vi "Convert-map-to-2D.vi"(8 "error in":errorcluster, 9 "Ycoords":sgl[](array[numeric]), 10 "Xcoords":sgl[](array[numeric]), 11 "Signal":dbl[](array[numeric])) -> (0 "error IO":errorcluster, 3 "2D map":dbl[][](array[numeric]))   [LabVIEW 2013, in "CameraVision.lvlib" / "CV-UI.lvclass"]
doc: "This function deletes the data from the various GUI graphs and displays. This avoids interference with data from a previous acquisition."
uses:
  CV-UI.lvclass
panel:
  out "Yscale":sgl
  out "Xscale":sgl
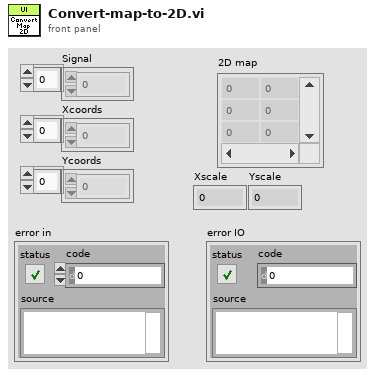
[diagram p1: front panel]
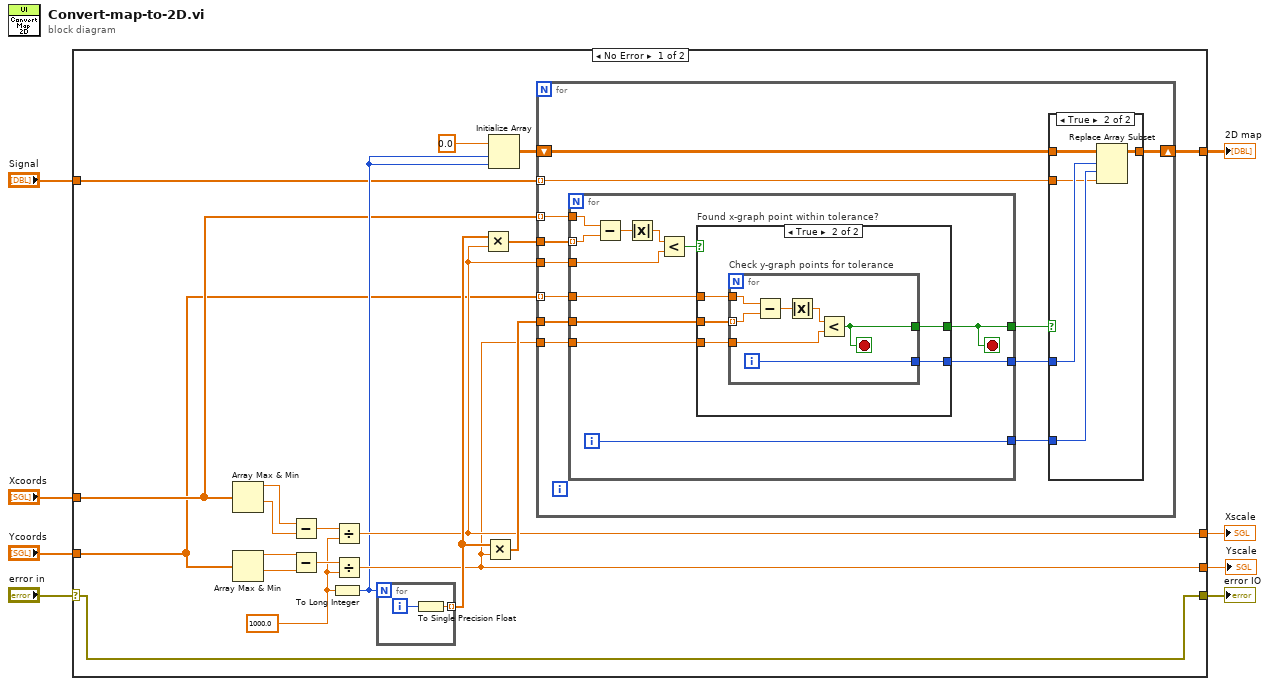
[diagram p0: block diagram]
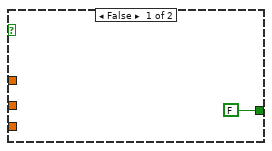
[diagram p3: hidden frame]
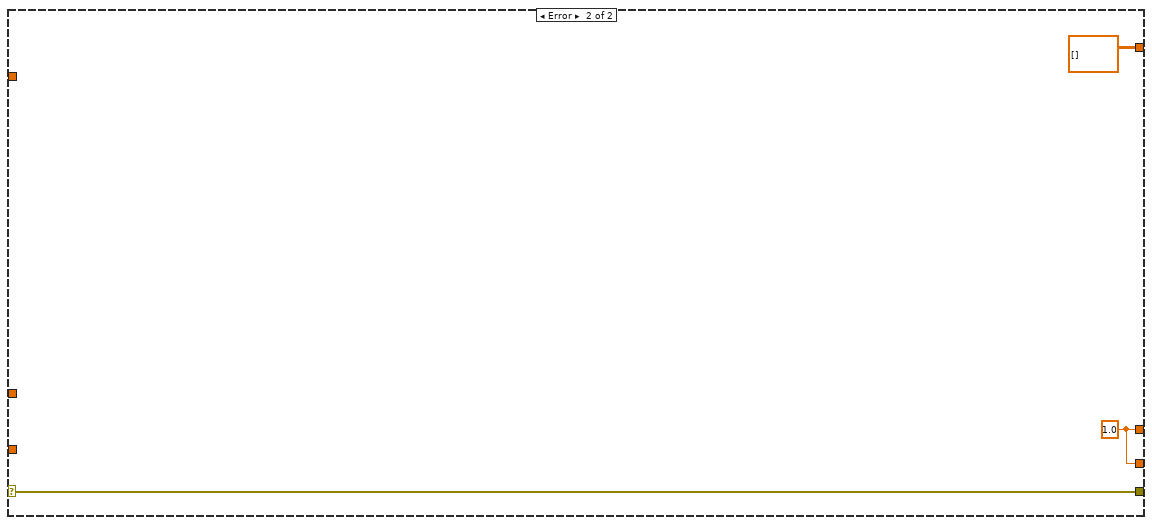
[diagram p4: hidden frame]
diagram:
  n1 = case shown="No Error" "error in" {
    selector: "error in" -> [w12 w76]
    tunnel: [w12 w76] -> w8
    tunnel: [w17 w75] -> w5
    tunnel: [w18 w75] -> w6
    tunnel: [w13 sgl[][] []] -> w4
    tunnel: "Xcoords" -> [w11 _]
    tunnel: "Ycoords" -> [w10 _]
    tunnel: "Signal" -> [w9 _]
    frame No Error {
      w22 = sgl 1000.0
      n2 = Array Max & Min(array=w11) -> (max value=w28:sgl, min value=w27:sgl)  [unwired: 2 out]
      n3 = Array Max & Min(array=w10) -> (max value=w24:sgl, min value=w23:sgl)  [unwired: 2 out]
      n4 = Subtract(x=w28, y=w27) -> (x-y=w25:sgl)
      n5 = Subtract(x=w24, y=w23) -> (x-y=w26:sgl)
      n6 = To Long Integer(number=w22) -> (32bit integer=w15:i32)
      n7 = Divide(x=w25, y=w22) -> (x/y=w18:sgl)
      n8 = Divide(x=w26, y=w22) -> (x/y=w17:sgl)
      n9 = for {
        N: w15 -> [_]
        tunnel: [w29] -> w20 mode=indexing
        i -> [w30]
        n10 = To Single Precision Float(number=w30) -> (single precision float=w29:sgl)
      }
      n11 = Multiply(x=w20, y=w18) -> (x*y=w19:sgl[])
      n12 = Multiply(x=w20, y=w17) -> (x*y=w21:sgl[])
      n13 = Initialize Array(0.0, w15, w15) -> (w14:dbl[][])
      n14 = for {
        tunnel: w21 -> [w39]
        tunnel: w19 -> [w42]
        tunnel: w11 -> [w41] mode=indexing
        tunnel: w18 -> [w40]
        tunnel: w17 -> [w38]
        tunnel: w10 -> [w37] mode=indexing
        tunnel: w9 -> [w31] mode=indexing
        shift-right: [w35] -> w13
        shift-left: w14 -> [w36]
        n15 = for {
          tunnel: w42 -> [w60] mode=indexing
          tunnel: w41 -> [w59]
          tunnel: w40 -> [w56]
          tunnel: w39 -> [w55]
          tunnel: w38 -> [w54]
          tunnel: [w52] -> w33
          tunnel: [w51] -> w34
          tunnel: [w50] -> w32
          tunnel: w37 -> [w49]
          i -> [w50]
          stop <- w51 stop-if-true
          n16 = Subtract(x=w59, y=w60) -> (x-y=w58:sgl)
          n17 = Absolute Value(x=w58) -> (abs(x)=w57:sgl)
          n18 = Less?(x=w57, y=w56) -> (x < y?=w53:bool)
          n19 = case "Found x-graph point within tolerance?" shown="True" w53 {
            tunnel: w55 -> [_ w66]
            tunnel: w54 -> [_ w65]
            tunnel: w49 -> [_ w64]
            tunnel: [FALSE w63] -> w51
            tunnel: [_ w62] -> w52
            frame False {
            }
            frame True {
              n20 = for "Check y-graph points for tolerance" {
                tunnel: w66 -> [w73] mode=indexing
                tunnel: w65 -> [w72]
                tunnel: w64 -> [w71]
                tunnel: [w68] -> w63
                tunnel: [w67] -> w62
                i -> [w67]
                stop <- w68 stop-if-true
                n21 = Subtract(x=w71, y=w73) -> (x-y=w70:sgl)
                n22 = Absolute Value(x=w70) -> (abs(x)=w69:sgl)
                n23 = Less?(x=w69, y=w72) -> (x < y?=w68:bool)
              }
            }
          }
        }
        n24 = case shown="True" w34 {
          tunnel: w36 -> [w43 w48]
          tunnel: [w43 w47] -> w35
          tunnel: w33 -> [_ w46]
          tunnel: w32 -> [_ w45]
          tunnel: w31 -> [_ w44]
          frame False {
          }
          frame True {
            n25 = Replace Array Subset(array=w48, new element=w44, index (row)=w46, index (col)=w45) -> (w47:dbl[][])
          }
        }
      }
    }
    frame Error {
      w75 = sgl 1.0
    }
  }
  "error IO" <- w8
  "2D map" <- w4
  "Xscale" <- w6
  "Yscale" <- w5
